vi "Test Function.vi"(11 "Error in":errorcluster) -> (15 "Error out":errorcluster)   [LabVIEW 2020, in "GetControlDetailsTests.lvlib"]
doc: "This VI validates the Panel A&B function"
uses:
  GetControlDetailsTests.lvlib
  <vilib>/Utility/Data Type/Type Definitions/Data Type.ctl
  <vilib>/addons/_JKI Toolkits/Caraya/classes/Test Suite/Define Test Suite (JUnit Report).vi
  <vilib>/SLL Drona/APIs/Stimulus/VI/MakeVIFrontMost.vi
  <vilib>/SLL Drona/APIs/Stimulus/ControlValue/SetValueAuto.vi
  <vilib>/SLL Drona/APIs/Assert/AssertControlValue/Equal.vi
  <vilib>/SLL Drona/APIs/Stimulus/VI/CloseVI.vi
  <vilib>/Utility/error.llb/Error Cluster From Error Code.vi
  <vilib>/ErrorRing/Error Ring.xnode
  <vilib>/addons/_JKI Toolkits/Caraya/classes/Test Suite/Test Suite.lvclass
  <vilib>/addons/_JKI Toolkits/Caraya/classes/Test/Test.lvclass
  <vilib>/SLL Drona/Drona.lvlib
  <vilib>/SLL Drona/APIs/Assert/AssertControlValue/AssertControlValue.lvlib
  <vilib>/Utility/Data Type/NI_Data Type.lvlib
  <vilib>/Wiresmith Technology/G CLI/CLI Class/CLI.lvclass
  <vilib>/SLL Drona/APIs/Stimulus/VI/VI.lvlib
  <vilib>/SLL Drona/APIs/Stimulus/ControlValue/ControlValue.lvlib
panel:
  # "PANEL A&B TEST"
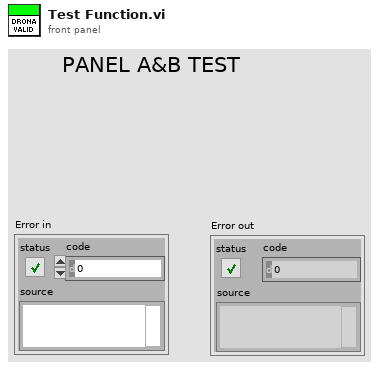
[diagram p1: front panel]
types:
  T1 = typedef "NI_Data Type.lvlib/Data Type.ctl" = enum8{"Invalid Type", "Void", "I8", "I16", "I32", "I64", "U8", "U16", "U32", "U64", "Single Float", "Double Float", "Extended Float", "Single Complex", "Double Complex", "Extended Complex", "Enum U8", "Enum U16", "Enum U32", "Enum U64", "Single Float With Unit", "Double Float With Unit", "Extended Float With Unit", "Single Complex with Unit", "Double Complex with Unit", "Extended Complex with Unit", "Boolean", "String", "Path", "Picture", "Tag", "Array", "Cluster", "Variant", "LV Variant", "Waveform", "Timestamp", "Digital Waveform", "Digital Data", "ExpressData", "Refnum", "External Data", "VI", "Poly VI", "LabVIEW Class Instance", "Fixed Point", "Set Collection", "Map Collection"}
  T2 = cluster{"type":T1, "Label.Text":string, "Visible":bool, "Value":variant}[]
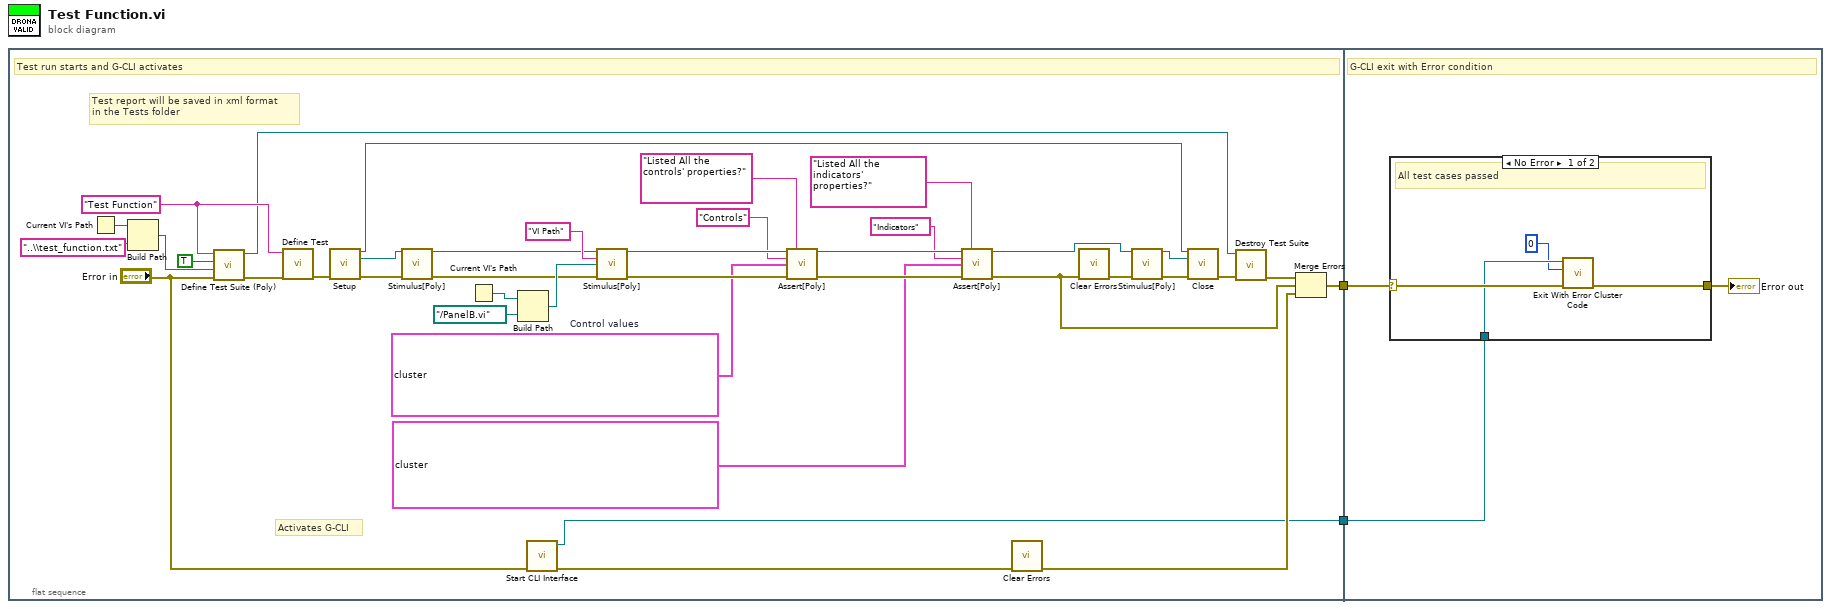
[diagram p0: block diagram]
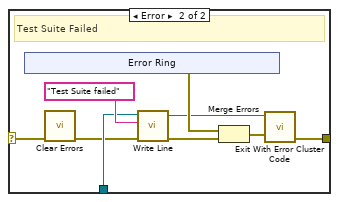
[diagram p2: hidden frame]
diagram:
  n1 = flat-sequence {
    tunnel: [w8] -> w2
    tunnel: [w7] -> w1
    tunnel: w2 -> [w44]
    tunnel: w1 -> [w43]
    frame #0 {
      w6 = T2 [{"type"=enum."Double Float", "Label.Text"="Numeric Control", "Visible"=TRUE, "Value"=variant(dbl 54.6)}, {"type"=enum."Boolean", "Label.Text"="Boolean Control", "Visible"=TRUE, "Value"=variant(bool TRUE)}, {"type"=enum."String", "Label.Text"="String Control", "Visible"=FALSE, "Value"=variant(string "ABCD34EFGH")}]  # Control values
      w21 = "Test Function" ("Label (VI Title)")
      # "Activates G-CLI"
      # "Test report will be saved in xml format\nin the Tests folder"
      # "Test run starts and G-CLI activates"
      n2 = Current VI's Path() -> (path=w20:path)
      n3 = Build Path(base path=w20, name or relative path="..\\test_function.txt") -> (appended path=w18:path)
      n4 = call-poly <vilib>:"Define Test Suite (Poly).vi"("error in (no error)"="Error in", "Report Path"=w18, "Interactive"=TRUE, "Label (VI Title)"=w21) -> ("error out"=w22:errorcluster, "Test Suite"=w15:refnum<class "Test Suite.lvclass">)  [unwired: 5 in, 1 out]
      n5 = call <vilib>:"Define Test.vi"("error in (no error)"=w22, "Label (VI Title)"=w21) -> ("error out"=w41:errorcluster)  [unwired: 8 in, 1 out]
      n6 = call <vilib>:"Setup.vi"("error in"=w41) -> ("Application Ref"=w29:refnum<vi>, "VI Reference Out"=w4:refnum<vi>, "error out"=w40:errorcluster)  [unwired: 12 in]
      n7 = call-poly <vilib>:"Stimulus[Poly].vi"("VI Reference In"=w4, "error in"=w40) -> ("VI Reference Out"=w3:refnum<vi>, "error out"=w5:errorcluster)  [unwired: 12 in]
      n8 = Current VI's Path() -> (path=w28:path)
      n9 = Build Path(base path=w28, name or relative path=path "../PanelB.vi") -> (appended path=w26:path)
      n10 = call <vilib>:"Start CLI Interface.vi"("error in (no error)"="Error in") -> ("error out"=w10:errorcluster, "CLI out"=w7:refnum<class "CLI.lvclass">)  [unwired: 7 in, 2 out]
      n11 = call-poly <vilib>:"Stimulus[Poly].vi"("VI Reference In"=w3, "Control Path"="VI Path", "Value (Signaling)"=w26, "error in"=w5) -> ("VI Reference Out"=w37:refnum<vi>, "error out"=w38:errorcluster)  [unwired: 10 in]
      n12 = call-poly <vilib>:"Assert[Poly].vi"("VI Reference In"=w37, "Test Label"="Listed All the controls' properties?" ("Label"), "Control Path"="Controls", "Control Value"=w6, "Error In"=w38) -> ("VI Reference Out"=w33:refnum<vi>, "Error Out"=w34:errorcluster)  [unwired: 9 in]
      n13 = call-poly <vilib>:"Assert[Poly].vi"("VI Reference In"=w33, "Test Label"="Listed All the indicators' properties?" ("Label"), "Control Path"="Indicators", "Control Value"=T2 [{"type"=enum."Double Float", "Label.Text"="Numeric Indicator", "Visible"=FALSE, "Value"=variant(dbl 54.6)}, {"type"=enum."Boolean", "Label.Text"="Boolean Indicator", "Visible"=TRUE, "Value"=variant(bool TRUE)}, {"type"=enum."String", "Label.Text"="String Indicator", "Visible"=TRUE, "Value"=variant(string "ABCD34EFGH")}] ("Indicator"), "Error In"=w34) -> ("VI Reference Out"=w25:refnum<vi>, "Error Out"=w11:errorcluster)  [unwired: 9 in]
      n14 = call <vilib>:"Clear Errors.vi"("error in (no error)"=w10) -> ("error out"=w9:errorcluster)  [unwired: 5 in, 1 out]
      n15 = call <vilib>:"Clear Errors.vi"("error in (no error)"=w11) -> ("error out"=w12:errorcluster)  [unwired: 5 in, 1 out]
      n16 = call-poly <vilib>:"Stimulus[Poly].vi"("VI Reference In"=w25, "error in"=w12) -> ("VI Reference Out"=w24:refnum<vi>, "error out"=w23:errorcluster)  [unwired: 12 in]
      n17 = call <vilib>:"Close.vi"("Application Ref"=w29, "VI Reference"=w24, "error in"=w23) -> ("error out"=w16:errorcluster)  [unwired: 12 in]
      n18 = call-dynamic "Destroy Test Suite.vi"("error in (no error)"=w16, "Test Suite in"=w15) -> ("error out"=w13:errorcluster)  [unwired: 8 in, 1 out]
      n19 = Merge Errors(w13, w11, w9) -> (w8:errorcluster)
    }
    frame #1 {
      # "G-CLI exit with Error condition"
      n20 = case shown="No Error" w44 {
        selector: w44 -> [w48 w52]
        tunnel: w43 -> [w47 w50]
        tunnel: [w45 w57] -> w42
        frame No Error {
          # "All test cases passed"
          n21 = call <vilib>:"Exit With Error Cluster Code.vi"("error in (no error)"=w48, "No Error Code (0)"=0, "CLI in"=w47) -> ("error out"=w45:errorcluster)  [unwired: 8 in]
        }
        frame Error {
          # "Test Suite Failed"
          n22 = xnode "Error Ring"() -> ("error out"=w54:errorcluster)
          n23 = call <vilib>:"Clear Errors.vi"("error in (no error)"=w52) -> ("error out"=w49:errorcluster)  [unwired: 5 in, 1 out]
          n24 = call <vilib>:"Write Line.vi"("error in (no error)"=w49, "Text to Write"="Test Suite failed", "CLI in"=w50) -> ("error out"=w53:errorcluster, "CLI out"=w51:refnum<class "CLI.lvclass">)  [unwired: 7 in]
          n25 = Merge Errors(w54, w53) -> (w55:errorcluster)
          n26 = call <vilib>:"Exit With Error Cluster Code.vi"("error in (no error)"=w55, "CLI in"=w51) -> ("error out"=w57:errorcluster)  [unwired: 9 in]
        }
      }
      "Error out" <- w42
    }
  }
